vi "Navx-Read (SubVI).vi"(8 "error in (no error)":errorcluster, 10 "I2C Ref Out":T1, 11 "Reset":bool) -> (0 "error out":errorcluster, 3 "PHI":dbl)   [LabVIEW 2017]
uses:
  <vilib>/myRIO/Instrument Drivers/Onboard IO/I2C/typedefs/I2C Reference.ctl
  <vilib>/myRIO/Common/Instrument Driver Framework/Utilities/typedefs/myRIO Generic Hardware Reference.ctl
  <vilib>/myRIO/Common/Instrument Driver Framework/Utilities/typedefs/Hardware Version Enum.ctl
  <vilib>/myRIO/Common/Instrument Driver Framework/Utilities/typedefs/myRIO v1.0 Reference.ctl
  <vilib>/myRIO/Common/Instrument Driver Framework/Utilities/typedefs/Generic FPGA Reference.ctl
  <vilib>/myRIO/Common/Instrument Driver Framework/myRIO v1.0/I2C/typedefs/I2C Channels Enum.ctl
  <vilib>/myRIO/Instrument Drivers/Onboard IO/I2C/typedefs/I2C Configuration.ctl
  <vilib>/myRIO/Instrument Drivers/Onboard IO/I2C/typedefs/I2C Transfer Rate.ctl
  <vilib>/Utility/error.llb/Error Cluster From Error Code.vi
  <vilib>/myRIO/Common/Instrument Driver Framework/myRIO v1.0/I2C/vis/myRIO v1.0 Write I2C.vi
  <vilib>/myRIO/Common/Instrument Driver Framework/myRIO v1.0/I2C/vis/myRIO v1.0 Read I2C.vi
  Projects/Auto control/Global 1.vi
  <vilib>/myRIO/Instrument Drivers/Onboard IO/I2C/I2C.lvlib
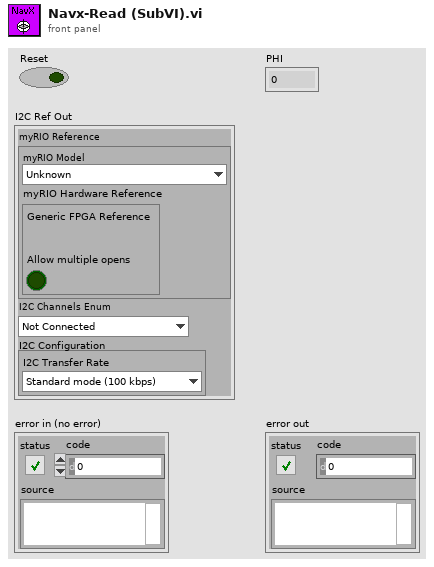
[diagram p1: front panel]
types:
  T1 = typedef "I2C.lvlib/I2C Reference.ctl" = cluster{"myRIO Reference":T2, "I2C Channels Enum":T6, "I2C Configuration":T7}
  T2 = typedef "myRIO Generic Hardware Reference.ctl" = cluster{"myRIO Model":T3, "myRIO Hardware Reference":T4}
  T3 = typedef "Hardware Version Enum.ctl" = enum16{"Unknown", "myRIO-1900", "myRIO-1950", "roboRIO", "NI ELVIS RIO CM"}
  T4 = typedef "myRIO v1.0 Reference.ctl" = cluster{"Generic FPGA Reference":T5, "Allow multiple opens":bool}
  T5 = typedef "Generic FPGA Reference.ctl" = refnum<k20>
  T6 = typedef "I2C Channels Enum.ctl" = enum16{"Not Connected", "A/I2C", "B/I2C", "I2C/I2C"}
  T7 = typedef "I2C.lvlib/I2C Configuration.ctl" = cluster{"I2C Transfer Rate":T8}
  T8 = typedef "I2C.lvlib/I2C Transfer Rate.ctl" = enum16{"Standard mode (100 kbps)", "Fast mode (400 kbps)"}
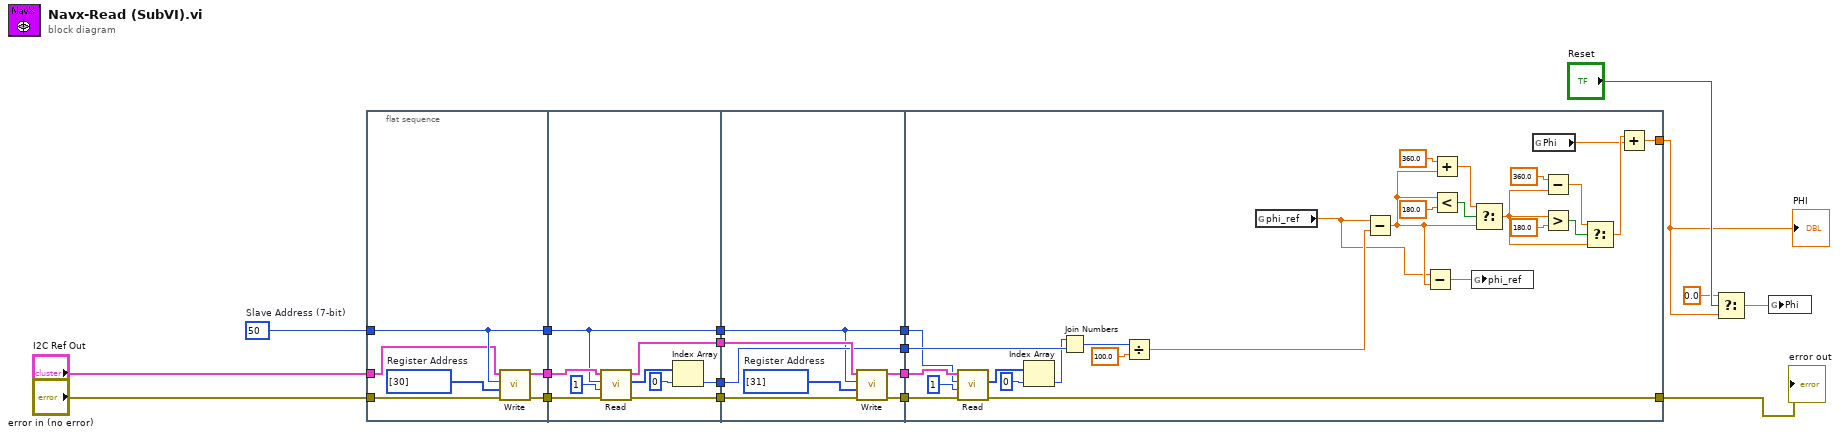
[diagram p0: block diagram]
diagram:
  w5 = u8 50  # Slave Address (7-bit)
  n1 = flat-sequence {
    tunnel: [w25] -> w16
    tunnel: [w24] -> w15
    tunnel: w5 -> [w22]
    tunnel: [w22] -> w14
    tunnel: "I2C Ref Out" -> [w21]
    tunnel: "error in (no error)" -> [w20]
    tunnel: w16 -> [w33]
    tunnel: w15 -> [w30]
    tunnel: w14 -> [w27]
    tunnel: [w29] -> w13
    tunnel: [w28] -> w12
    tunnel: [w27] -> w11
    tunnel: [w26] -> w10
    tunnel: w13 -> [w40]
    tunnel: w12 -> [w39]
    tunnel: w11 -> [w35]
    tunnel: [w38] -> w9
    tunnel: [w37] -> w8
    tunnel: [w36] -> w7
    tunnel: w10 -> [w36]
    tunnel: [w35] -> w6
    tunnel: w9 -> [w65]
    tunnel: w8 -> [w64]
    tunnel: [w63] -> w19
    tunnel: w7 -> [w62]
    tunnel: w6 -> [w60]
    tunnel: [w47] -> w2
    frame #0 {
      w23 = u8[] [30]  # Register Address
      n2 = call <vilib>:"Write.vi"("error in (no error)"=w20, "Bytes to Write"=w23, "Slave Address (7-bit)"=w22, "I2C Ref In"=w21) -> ("error out"=w24:errorcluster, "I2C Ref Out"=w25:T1)  [unwired: 6 in]
    }
    frame #1 {
      n3 = call <vilib>:"Read.vi"("error in (no error)"=w30, "Byte Count"=u32 1, "Slave Address (7-bit)"=w27, "I2C Ref In"=w33) -> ("error out"=w28:errorcluster, "Bytes Read"=w32:u8[], "I2C Ref Out"=w29:T1)  [unwired: 4 in]
      n4 = Index Array(array=w32, index=0) -> (element=w26:u8)
    }
    frame #2 {
      w41 = u8[] [31]  # Register Address
      n5 = call <vilib>:"Write.vi"("error in (no error)"=w39, "Bytes to Write"=w41, "Slave Address (7-bit)"=w35, "I2C Ref In"=w40) -> ("error out"=w37:errorcluster, "I2C Ref Out"=w38:T1)  [unwired: 6 in]
    }
    frame #3 {
      n6 = call <vilib>:"Read.vi"("error in (no error)"=w64, "Byte Count"=u32 1, "Slave Address (7-bit)"=w60, "I2C Ref In"=w65) -> ("error out"=w63:errorcluster, "Bytes Read"=w67:u8[])  [unwired: 4 in, 1 out]
      n7 = Index Array(array=w67, index=0) -> (element=w61:u8)
      n8 = Join Numbers(hi=w61, lo=w62) -> ((hi.lo)=w58:u16)
      n9 = Divide(x=w58, y=100.0) -> (x/y=w46:dbl)
      n10 = global read "Global 1.vi" "phi_ref"() -> (w44:dbl)
      n11 = Subtract(x=w44, y=w46) -> (x-y=w45:dbl)
      n12 = Subtract(x=w44, y=w45) -> (x-y=w43:dbl)
      n13 = Add(x=360.0, y=w45) -> (x+y=w49:dbl)
      n14 = Less?(x=w45, y=180.0) -> (x < y?=w51:bool)
      n15 = global write "Global 1.vi" "phi_ref"(w43) -> ()
      n16 = Select(t=w49, s=w51, f=w45) -> (s? t:f=w48:dbl)
      n17 = global read "Global 1.vi" "Phi"() -> (w42:dbl)
      n18 = Subtract(x=360.0, y=w48) -> (x-y=w54:dbl)
      n19 = Greater?(x=w48, y=180.0) -> (0:w56:bool)
      n20 = Select(t=w54, s=w56, f=w48) -> (s? t:f=w53:dbl)
      n21 = Add(x=w53, y=w42) -> (x+y=w47:dbl)
    }
  }
  n22 = Select(t=0.0, s="Reset", f=w2) -> (s? t:f=w1:dbl)
  n23 = global write "Global 1.vi" "Phi"(w1) -> ()
  "PHI" <- w2
  "error out" <- w19
